vi "SetValueWidth.vi"(8 "error in (no error)":errorcluster, 10 "Value Width":enum16{"4-bit", "8-bit"}(ring), 11 "ControlState in":T1 {"ChainMask" format="0x%02x"}) -> (0 "error out":errorcluster, 3 "ControlState out":T1 {"ChainMask" format="0x%02x"})   [LabVIEW 2023, in "ArduinoSerialBling.lvlib"]
uses:
  ArduinoSerialBling.lvlib
  ControlState.ctl
  ConnectionType.ctl
  UdpConnection.ctl
  ChainState.ctl
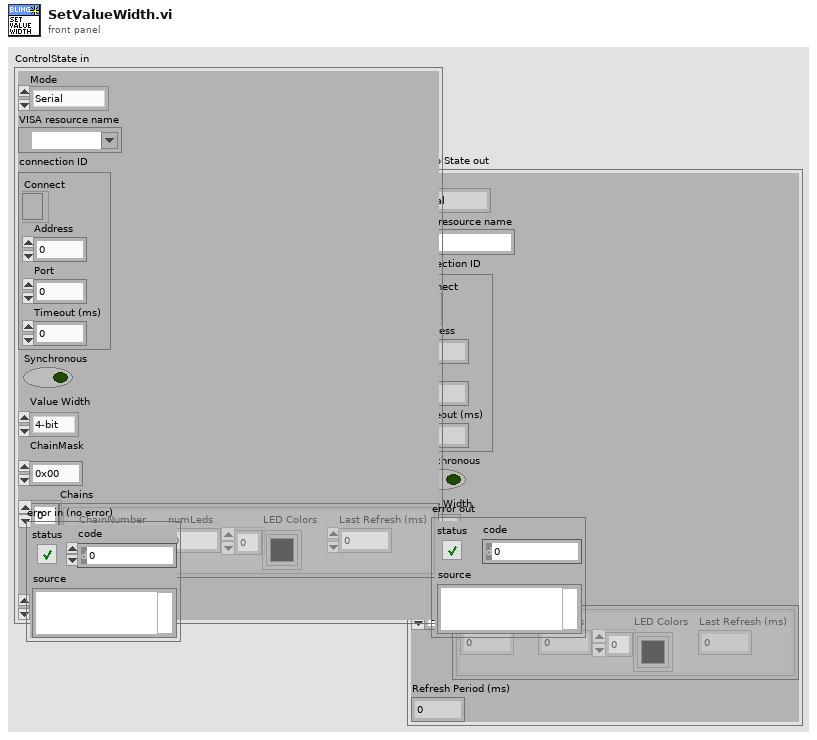
[diagram p1: front panel]
types:
  T1 = typedef "ArduinoSerialBling.lvlib/ControlState.ctl" = cluster{"Mode":T2, "VISA resource name":refnum<visa-resource-name>, "connection ID":T3, "Synchronous":bool, "Value Width":enum16{"4-bit", "8-bit"}, "ChainMask":u8, "Chains":T4[], "Refresh Period (ms)":u32}
  T2 = typedef "ConnectionType.ctl" = enum16{"Serial", "Ethernet", "Offline"}
  T3 = typedef "UdpConnection.ctl" = cluster{"Connect":refnum<k16>, "Address":u32, "Port":u16, "Timeout (ms)":i32}
  T4 = typedef "ArduinoSerialBling.lvlib/ChainState.ctl" = cluster{"ChainNumber":u8, "numLeds":u8, "LED Colors":u32[], "Last Refresh (ms)":u32}
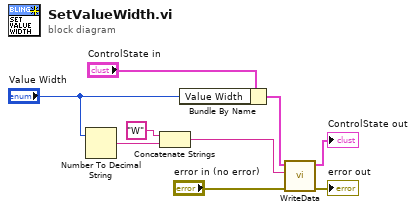
[diagram p0: block diagram]
diagram:
  n1 = Number To Decimal String(number="Value Width") -> (decimal integer string=w7:string)  [unwired: 1 in]
  n2 = Concatenate Strings("W", w7) -> (w4:string)
  n3 = Bundle By Name(cluster="ControlState in", "Value Width"="Value Width") -> (w2:T1)
  n4 = call "WriteData.vi"("error in (no error)"="error in (no error)", "Command"=w4, "ControlState in"=w2) -> ("error out"=→"error out":errorcluster, "ControlState out"=→"ControlState out":T1)  [unwired: 5 in, 2 out]
